vi "Send Start Polling Msg.vi"(8 "error in (no error)":errorcluster, 10 "Message to Repeat":refnum<class "~Message.lvclass">, 11 "Message Queue":refnum<queue>) -> (0 "error out":errorcluster, 3 "Message Queue":refnum<queue>)   [LabVIEW 2024, in "Zero Timeout Message Handler.lvlib" / "Start Polling Msg.lvclass"]
uses:
  Start Polling Msg.lvclass
  Start Polling Msg.lvclass/Start Polling Msg.ctl
  ~Message/~Message.lvclass
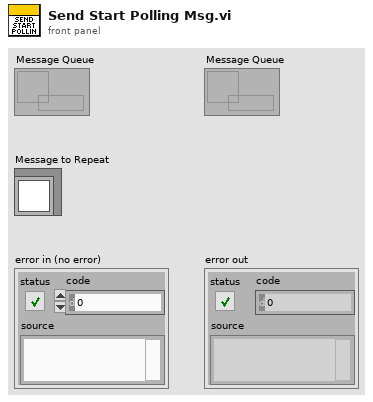
[diagram p1: front panel]
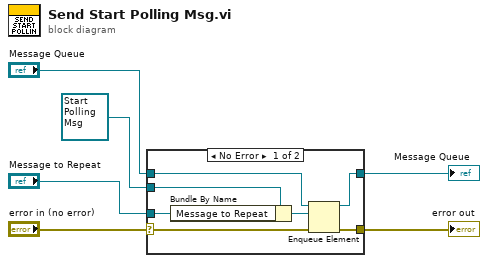
[diagram p0: block diagram]
diagram:
  n1 = case shown="No Error" "error in (no error)" {
    selector: "error in (no error)" -> [w11 w15]
    tunnel: "Message Queue" -> [w13 w14]
    tunnel: [w12 w15] -> w5
    tunnel: refnum<class "Start Polling Msg.lvclass"> refnum ("Zero Timeout Message Handler.lvlib:Start Polling Msg.lvclass") -> [w9 _]
    tunnel: [w10 w14] -> w2
    tunnel: "Message to Repeat" -> [w7 _]
    frame No Error {
      n2 = Bundle By Name(cluster=w9, "Message to Repeat"=w7) -> (w8:refnum<class "Start Polling Msg.lvclass">)
      n3 = Enqueue Element(queue=w13, element=w8, error in (no error)=w11) -> (queue out=w10:refnum<queue>, error out=w12:errorcluster)  [unwired: 1 in, 1 out]
    }
    frame Error {
    }
  }
  "error out" <- w5
  "Message Queue" <- w2
